vi "曲线平滑.vi"(10 "测量":cluster{dbl[], dbl[]}, 11 "理论":cluster{dbl[], dbl[]}) -> (1 "确认修改":bool, 2 "实测":cluster{dbl[], dbl[]}, 3 "理论":cluster{dbl[], dbl[]})   [LabVIEW 2015]
uses:
  <vilib>/Analysis/3filter.llb/Filter Passband Type.ctl
  <vilib>/Analysis/3filter.llb/Butterworth Filter (DBL).vi
  <vilib>/Analysis/NI_AALBase.lvlib
panel:
  in  "滤波频率":dbl=0.12500000000000006 caption="低通频率" min=0.0 format="%0.4f"
  in  "采样间隔":dbl=1.0 min=0.0 format="%0.2f"
  out "XY图":cluster{dbl[], dbl[]}[](graph)
  in  "取消":bool
  in  "确定":bool
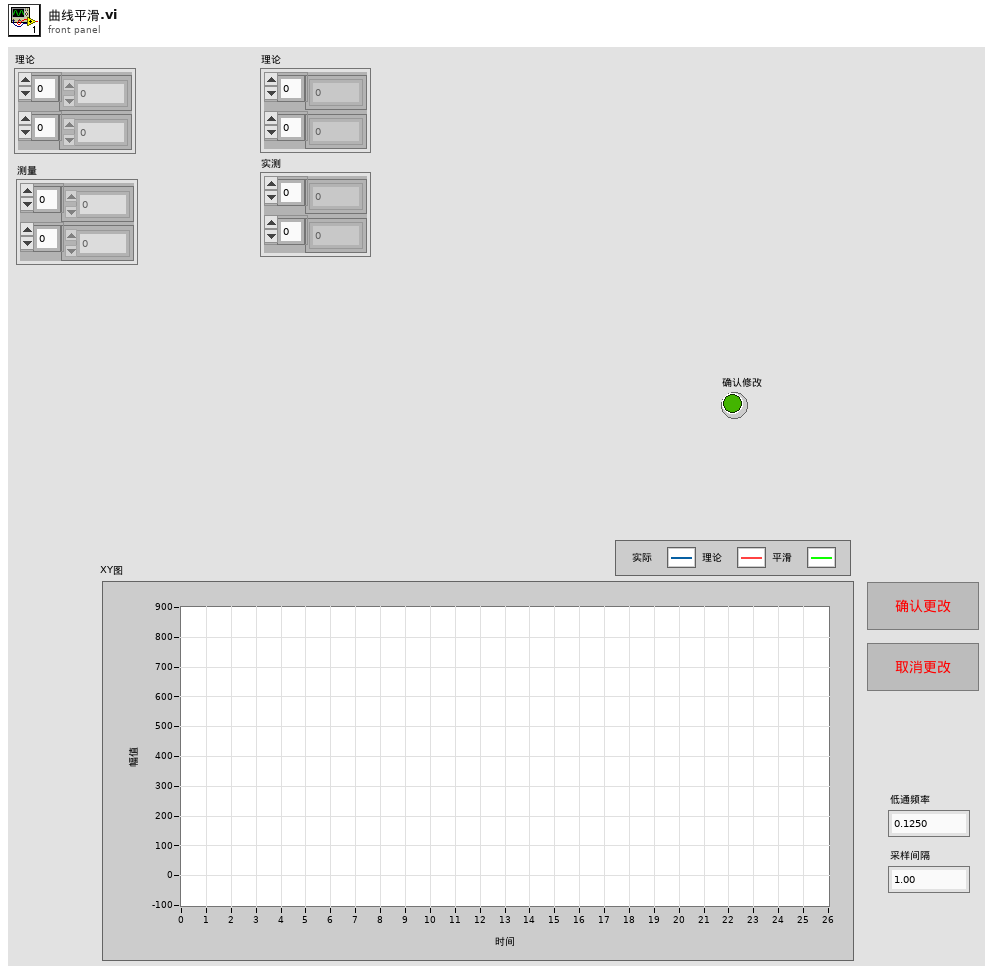
[diagram p1: front panel]
types:
  T1 = typedef "NI_AALBase.lvlib/Filter Passband Type.ctl" = enum32{"Lowpass", "Highpass", "Bandpass", "Bandstop"}
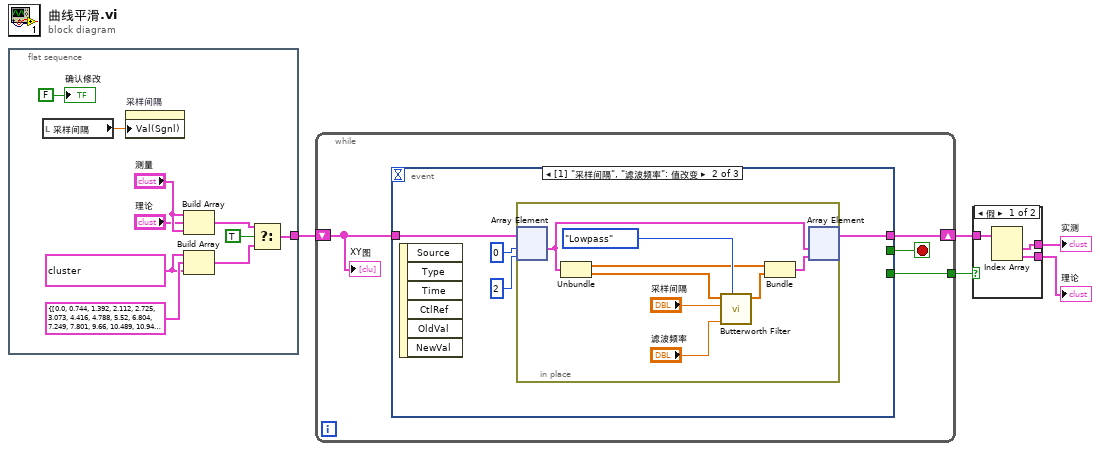
[diagram p0: block diagram]
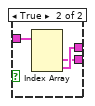
[diagram p2: hidden frame]
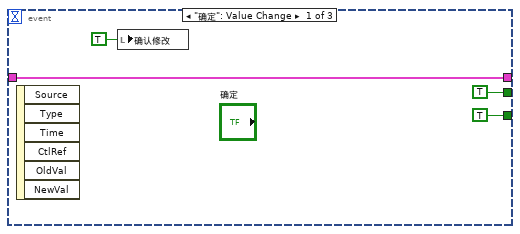
[diagram p3: hidden frame]
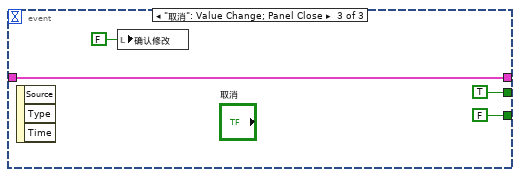
[diagram p4: hidden frame]
diagram:
  n1 = flat-sequence {
    tunnel: [w14] -> w2
    frame #0 {
      w11 = cluster{dbl[], dbl[]} {array[779 elements], array[779 elements]}
      n2 = local read "采样间隔"() -> (w7:dbl)
      n3 = property on="采样间隔" class="DigNum (严格)"("Val(Sgnl)"=w7) -> ()  [unwired: 2 in, 2 out]
      n4 = Build Array("测量", "理论", "测量") -> (w13:cluster{dbl[], dbl[]}[])
      n5 = Build Array(w11, cluster{dbl[], dbl[]} {[0.0, 0.744, 1.392, 2.112, 2.725, 3.073, 4.416, 4.788, 5.52, 6.804, 7.249, 7.801, 9.66, 10.489, 10.944, 11.341, 11.676, 11.988, 14.628, 15.288, 16.056, 16.821, 17.653], [0.0, 84.0, 194.0, 425.0, 493.0, 442.0, 431.0, 313.0, 395.0, 307.0, 263.0, 367.0, 309.0, 272.0, 259.0, 307.0, 310.0, 322.0, 408.0, 578.0, 803.0, 596.0, 0.0]}, w11) -> (w10:cluster{dbl[], dbl[]}[])
      n6 = Select(t=w13, s=TRUE, f=w10) -> (s? t:f=w14:cluster{dbl[], dbl[]}[])
      "确认修改" <- FALSE ("确认修改")
    }
  }
  n7 = while {
    shift-right: [w18] -> w5
    shift-left: w2 -> [w16]
    tunnel: [w17] -> w1
    stop <- w19 stop-if-true
    n8 = event shown="[1] \"采样间隔\", \"滤波频率\": 值改变" {
      selector: _ -> [_ _ _]
      dyn-events: _ -> [_ _ _]
      timeout: _ -> [_ _ _]
      tunnel: [TRUE _ TRUE] -> w19
      tunnel: w16 -> [w23 w27 w38]
      tunnel: [w23 w25 w38] -> w18
      tunnel: [TRUE _ FALSE] -> w17
      event "确定": Value Change {
        n9 = event-data() -> ()  [unwired: 1 in, 6 out]
        n10 = local write "确认修改"(TRUE ("确认修改")) -> ()
      }
      event "采样间隔", "滤波频率": Value Change {
        n11 = event-data() -> ()  [unwired: 1 in, 6 out]
        n12 = in-place {
          n13 = in-place-array #1(w27, 0, 2) -> (w28:cluster{dbl[], dbl[]})  [unwired: 1 out]
          n14 = Unbundle(w28) -> (w31:dbl[], w32:dbl[])
          n15 = call-poly <vilib>:"Butterworth Filter.vi"("filter type"=Filter_Passband_Type."Lowpass", "low cutoff freq: fl"="滤波频率", "sampling freq: fs"="采样间隔", "X"=w32) -> ("Filtered X"=w30:dbl[])  [unwired: 4 in, 1 out]
          n16 = Bundle(w31, "Filtered X"=w30) -> (w29:cluster{dbl[], "Filtered X":dbl[]})  [unwired: 1 in]
          n17 = in-place-array #1(w28, w29) -> (w25:cluster{dbl[], dbl[]}[])  [unwired: 2 out]
        }
      }
      event "取消": Value Change; Panel Close {
        n18 = event-data() -> ()  [unwired: 1 in, 3 out]
        n19 = local write "确认修改"(FALSE ("确认修改")) -> ()
      }
    }
    "XY图" <- w16
  }
  n20 = case shown="假" w1 {
    tunnel: w5 -> [w42 w45]
    tunnel: [w40 w43] -> w4
    tunnel: [w41 w44] -> w3
    frame False {
      n21 = Index Array(array=w42) -> (element #1=w41:cluster{dbl[], dbl[]}, element #2=w40:cluster{dbl[], dbl[]})  [unwired: 2 in]
    }
    frame True {
      n22 = Index Array(array=w45) -> (element #2=w43:cluster{dbl[], dbl[]}, element #3=w44:cluster{dbl[], dbl[]})  [unwired: 3 in, 1 out]
    }
  }
  "理论" <- w4
  "实测" <- w3
